vi "Move_Trav_while_Meas_Blocks.vi"() -> (5 "Plug in titles":string[](array[string]), 7 "Plug in values":string[](array[string]))   [LabVIEW 2022 SP3]
uses:
  Controls/Post_Process.ctl
  Controls/Setup.ctl
  Gen Trav/Trav_mode.ctl
  Controls/User_Specific_mode.ctl
  Controls/Tunnel_Coordinates.ctl
  Globals/Trav_pos_global.vi
  Globals/Meas_global.vi
panel:
  in  "2nd delay":u32=6000
  out "Speed Factor":sgl=2.0 min=0.01 max=15 format="%.2f"
  in  "Delay between Rendezvous and Acquisition starting (ms)":u32
  in  "1st delay":u32=2000
  out "Case Currently On":string="Reset Traverse Speed Factor"
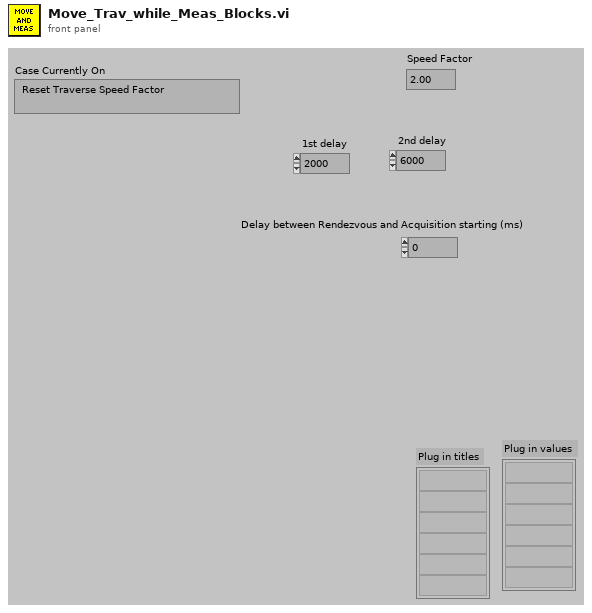
[diagram p1: front panel]
types:
  T1 = typedef "Traverse_cluster.ctl" = cluster{"Start X":sgl, "Start Y":sgl, "Start Z":sgl, "End X":sgl, "End Y":sgl, "End Z":sgl, "nPoints":i32, "Spacing":T2, "Filename":path, "Tunnel Speed":dbl, "Averaging time (mins)":dbl, "Extra Commands":string, "Carrier_1 Q (l/min)":dbl, "Carrier_2 Q (l/min)":dbl, "Trace Gas Concentration (%)":dbl, "Specific Arguments":string, "Comments":string, "Row No":i32, "Row Type Selector":T3, "EstCompl":string, "Row Duration (mins)":dbl, "nValidPoints":i32, "Meas Setup File":string}
  T2 = typedef "Spacing.ctl" = enum16{"Linear", "Log", "Gauss", "Specified", "N/A"}
  T3 = typedef "Multi_run_mode.ctl" = enum16{"Move Traverse Only", "Set Tunnel Speed Only", "Set Source Only", "Set Measurement Conditions", "Single Measurement", "Vertical Profile", "Lateral Profile", "Longitudinal Profile", "Multi-Axis Profile", "Explore Volume", "Auto Calibrate", "Meas Fast FID Bkgnd", "Check Beam Power", "Scanning Valve Measurement", "Run VI Named:", "Set ADAM Ch", "Wait (minutes)", "Send Message", "Synchronize With:", "Fall Back to this Row", "Turn Off Row Repeating", "Traverse 3D Volume", "Blank Row", "Jump to Fall Back Row"}
  T4 = typedef "Setup.ctl" = enum16{"Run Program", "Show Setup", "Save Current Setup", "Setup Front Panel"}
  T5 = typedef "Post_Process.ctl" = enum16{"Take New Data", "Post Process Raw Data File"}
  T6 = typedef "Tunnel_Coordinates.ctl" = enum16{"Work in Tunnel Coordinates", "Work in Model Coordinates"}
  T7 = typedef "User_Specific_mode.ctl" = enum16{"Check VI only", "Run VI"}
  T8 = typedef "Trav_mode.ctl" = enum16{"Move traverse", "Read traverse position", "Teach Position"}
  T9 = typedef "Rendezvous RefNum" = refnum<k1>
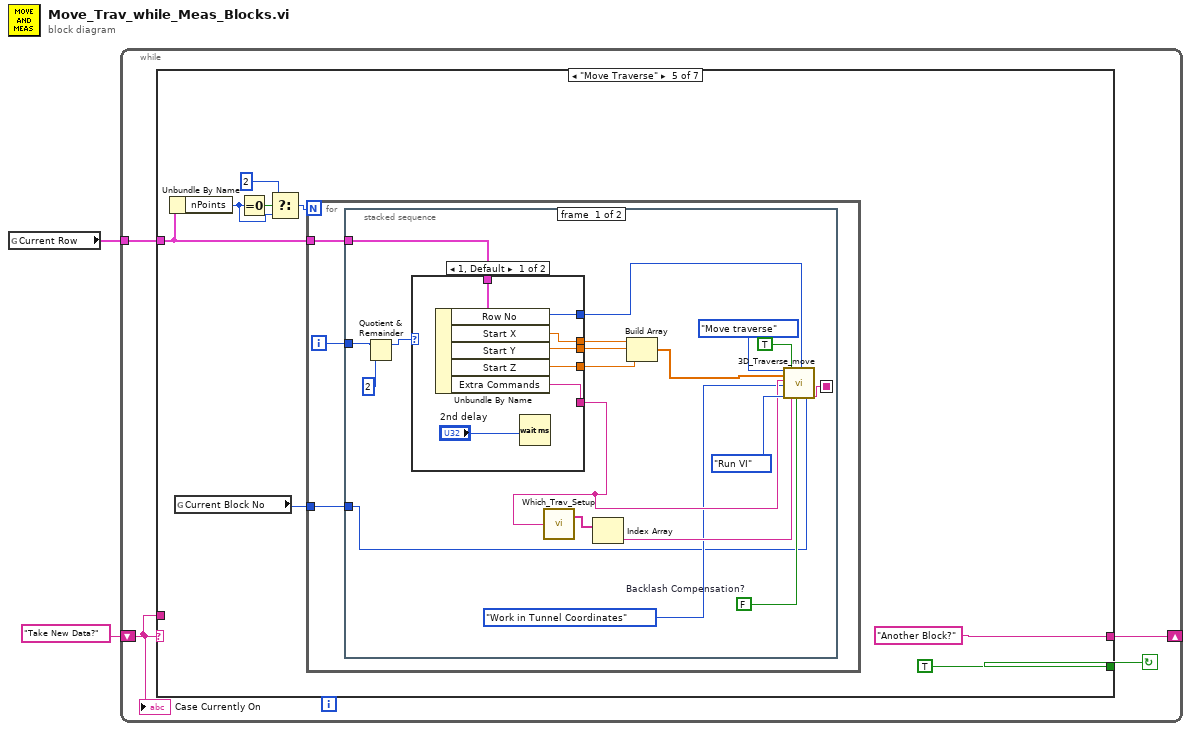
[diagram p0: block diagram]
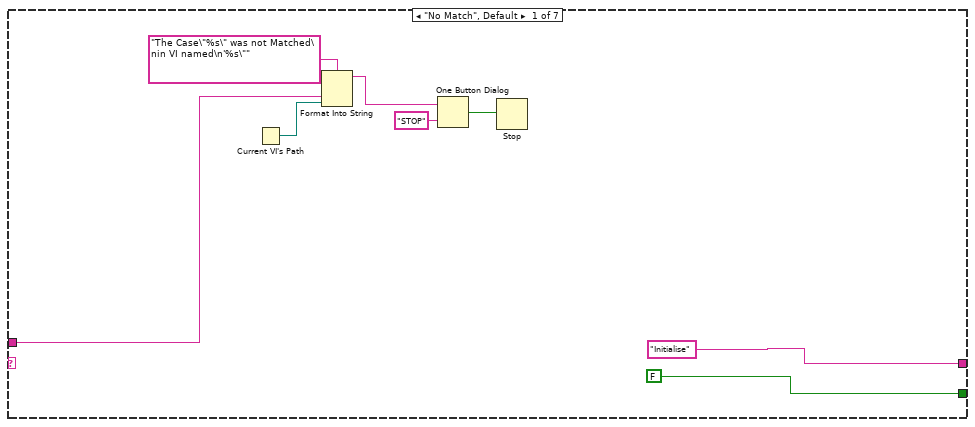
[diagram p2: hidden frame]
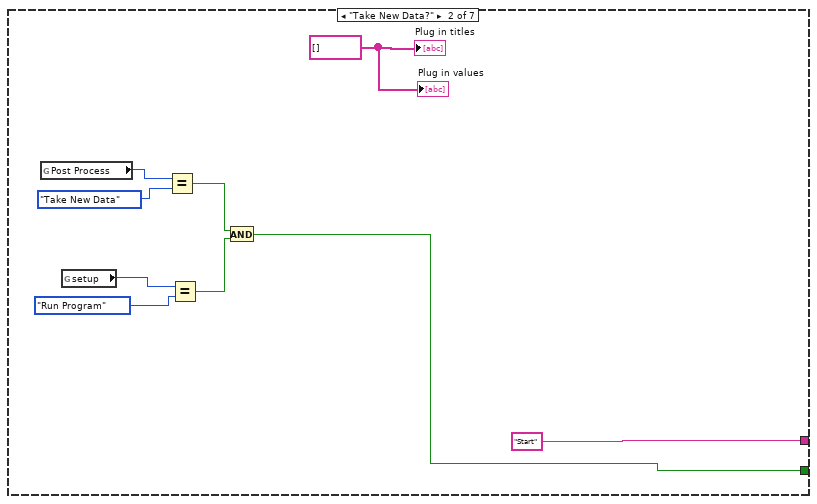
[diagram p3: hidden frame]
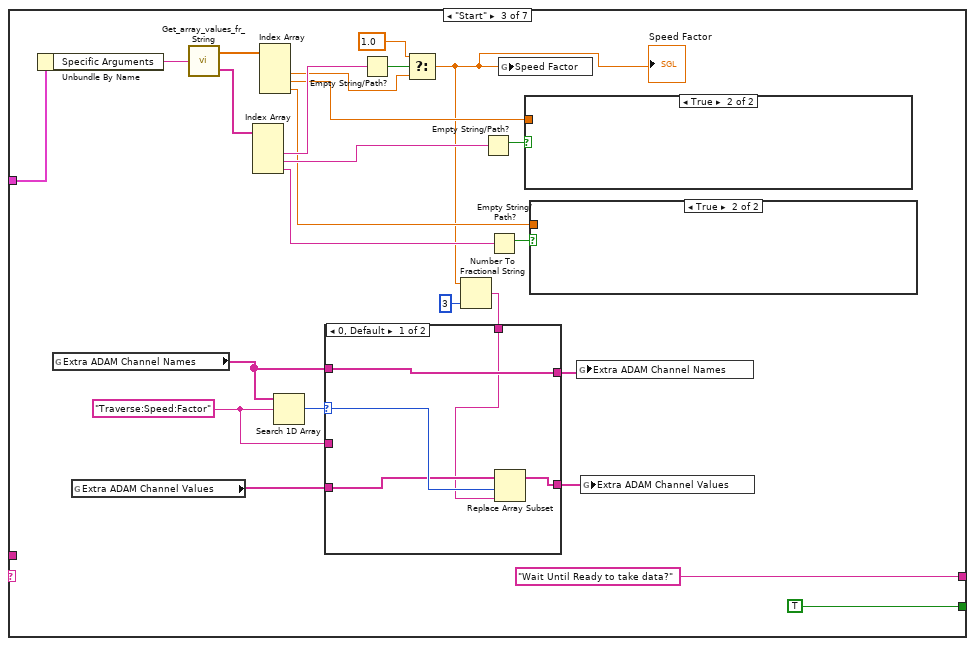
[diagram p4: hidden frame]
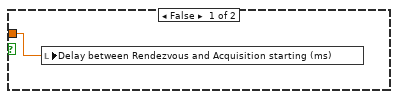
[diagram p5: hidden frame]
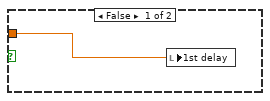
[diagram p6: hidden frame]
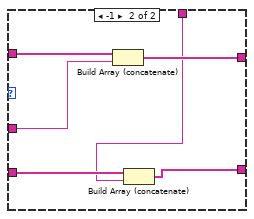
[diagram p7: hidden frame]
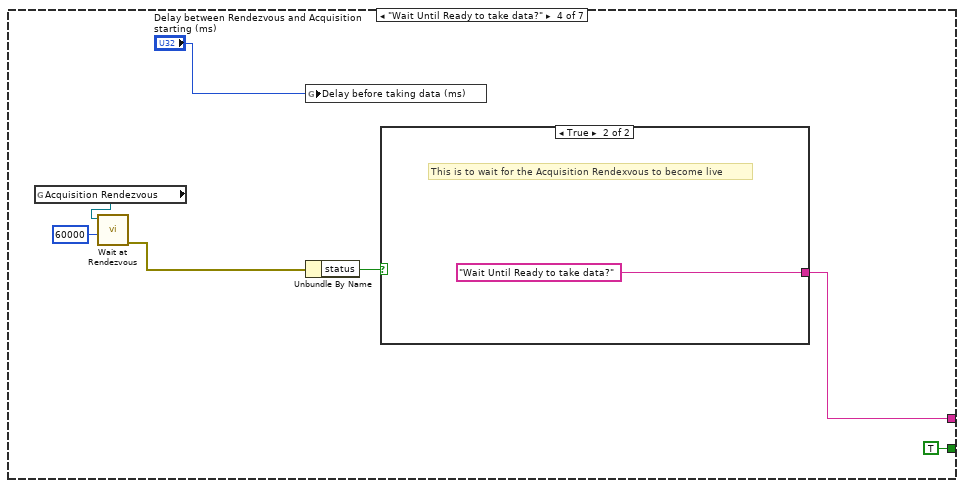
[diagram p8: hidden frame]
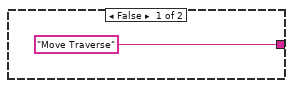
[diagram p9: hidden frame]
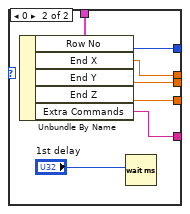
[diagram p10: hidden frame]
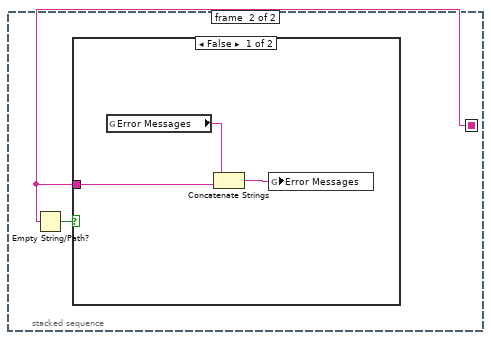
[diagram p11: hidden frame]
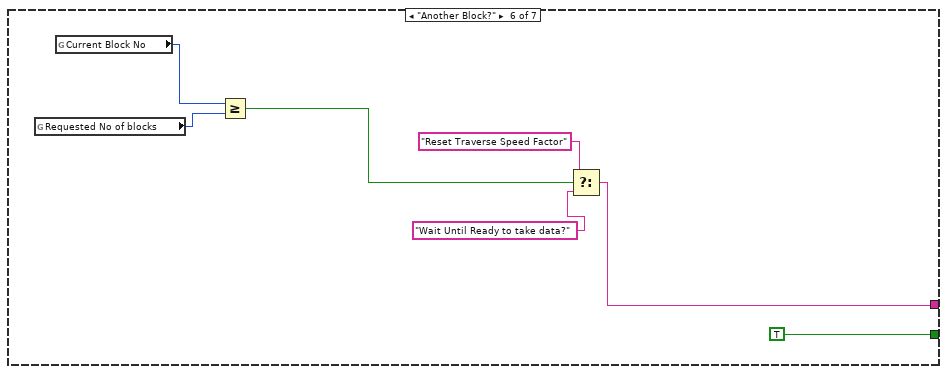
[diagram p13: hidden frame]
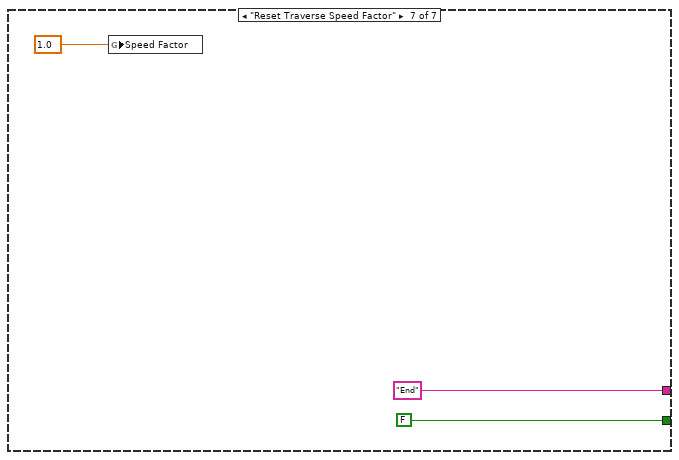
[diagram p14: hidden frame]
diagram:
  n1 = global read "Trav_pos_global.vi" "Current Row"() -> (w1:T1)
  n2 = while {
    shift-left: "Take New Data?" -> [w4]
    shift-right: [w5] -> _
    tunnel: w1 -> [w3]
    stop <- w6 continue-if-true
    n3 = case shown="\"Move Traverse\"" w4 {
      tunnel: [FALSE w15 TRUE ("Command Found") TRUE ("Command Found") TRUE ("Command Found") TRUE ("Command Found") FALSE ("Command Found")] -> w6
      tunnel: ["Initialise" "Start" "Wait Until Ready to take data?" ("f") w64 "Another Block?" w122 "End" ("f")] -> w5
      tunnel: w4 -> [w9 _ _ _ _ _ _]
      tunnel: w3 -> [_ _ w46 _ w75 _ _]
      frame "No Match", Default {
        n4 = Current VI's Path() -> (path=w8:path)
        n5 = Format Into String(format string="The Case\"%s\" was not Matched\nin VI named\n'%s\"" ("Format String"), w9, w8) -> (resulting string=w12:string)  [unwired: 2 in, 1 out]
        n6 = One Button Dialog(message=w12, button name ("OK")="STOP") -> (true=w10:bool)
        n7 = Stop(stop? (T)=w10) -> ()
      }
      frame "Take New Data?" {
        w20 = string[] [] ("Plug in titles")
        n8 = global read "Meas_global.vi" "Post Process"() -> (w22:T5)
        n9 = global read "Meas_global.vi" "setup"() -> (w19:T4)
        n10 = Equal?(x=w22, y=Post_Process."Take New Data" ("Post Process")) -> (x = y?=w16:bool)
        n11 = Equal?(x=w19, y=Setup."Run Program" ("setup")) -> (x = y?=w17:bool)
        n12 = And(x=w16, y=w17) -> (x .and. y?=w15:bool)
        "Plug in titles" <- w20
        "Plug in values" <- w20
      }
      frame "Start" {
        w36 = "Traverse:Speed:Factor"
        n13 = Unbundle By Name(w46) -> ("Specific Arguments"=w48:string)
        n14 = global read "Meas_global.vi" "Extra ADAM Channel Names"() -> (w37:string[])
        n15 = global read "Meas_global.vi" "Extra ADAM Channel Values"() -> (w34:string[])
        n16 = call "Get_array_values_fr_String.vi"("String Value"=w48) -> ("Numeric Array"=w47:dbl[], "String array"=w45:string[])
        n17 = Index Array(array=w45) -> (element #2=w44:string, element #3=w31:string, element #4=w27:string)  [unwired: 4 in, 1 out]
        n18 = Index Array(array=w47) -> (element #2=w42:dbl, element #3=w29:dbl, element #4=w25:dbl)  [unwired: 4 in, 1 out]
        n19 = Search 1D Array(1D array=w37, element=w36) -> (index of element=w38:i32)  [unwired: 1 in]
        n20 = Empty String/Path?(string/path=w44) -> (empty?=w43:bool)
        n21 = Select(t=1.0, s=w43, f=w42) -> (s? t:f=w24:dbl)
        "Speed Factor" <- w24
        n22 = Number To Fractional String(number=w24, precision (6)=i16 3) -> (F-format string=w28:string)  [unwired: 2 in]
        n23 = case shown="0, Default" w38 {
          selector: w38 -> [w54 _]
          tunnel: w37 -> [w55 w61]
          tunnel: w36 -> [_ w60]
          tunnel: [w55 w59] -> w35
          tunnel: w34 -> [w53 w58]
          tunnel: [w52 w57] -> w33
          tunnel: w28 -> [w51 w56]
          frame 0, Default {
            n24 = Replace Array Subset(array=w53, new element=w51, index=w54) -> (w52:string[])
          }
          frame -1 {
            n25 = Build Array (concatenate)(w61, w60) -> (w59:string[])
            n26 = Build Array (concatenate)(w58, w56) -> (w57:string[])
          }
        }
        n27 = Empty String/Path?(string/path=w31) -> (empty?=w30:bool)
        n28 = Empty String/Path?(string/path=w27) -> (empty?=w26:bool)
        n29 = global write "Trav_pos_global.vi" "Speed Factor"(w24) -> ()
        n30 = case shown="True" w30 {
          tunnel: w29 -> [w50 _]
          frame False {
            n31 = local write "1st delay"(w50) -> ()
          }
          frame True {
          }
        }
        n32 = case shown="True" w26 {
          tunnel: w25 -> [w49 _]
          frame False {
            n33 = local write "Delay between Rendezvous and Acquisition starting (ms)"(w49) -> ()
          }
          frame True {
          }
        }
        n34 = global write "Meas_global.vi" "Extra ADAM Channel Names"(w35) -> ()
        n35 = global write "Meas_global.vi" "Extra ADAM Channel Values"(w33) -> ()
      }
      frame "Wait Until Ready to take data?" {
        n36 = global read "Meas_global.vi" "Acquisition Rendezvous"() -> (w67:T9)
        n37 = call <vilib>:"Wait at Rendezvous.vi"("ms timeout (-1)"=60000, "rendezvous"=w67) -> ("error out"=w66:errorcluster)  [unwired: 3 in, 2 out]
        n38 = global write "Meas_global.vi" "Delay before taking data (ms)"("Delay between Rendezvous and Acquisition starting (ms)") -> ()
        n39 = Unbundle By Name(w66) -> ("status"=w63:bool)
        n40 = case shown="True" w63 {
          tunnel: ["Move Traverse" "Wait Until Ready to take data?"] -> w64
          frame False {
          }
          frame True {
            # "This is to wait for the Acquisition Rendexvous to become live"
          }
        }
      }
      frame "Move Traverse" {
        n41 = Unbundle By Name(w75) -> ("nPoints"=w72:i32)
        n42 = global read "Meas_global.vi" "Current Block No"() -> (w76:i32)
        n43 = Equal To 0?(x=w72) -> (x = 0?=w74:bool)
        n44 = Select(t=2, s=w74, f=w72) -> (s? t:f=w73:i32)
        n45 = for {
          N: w73 -> [_]
          tunnel: w75 -> [w81]
          tunnel: w76 -> [w80]
          i -> [w79]
          n46 = stacked-sequence {
            seq-local: [w85 _] -> [_ w115]
            tunnel: w81 -> [w92 _]
            tunnel: w80 -> [w86 _]
            tunnel: w79 -> [w83 _]
            frame #0 {
              w100 = FALSE  # Backlash Compensation?
              n47 = Quotient & Remainder(x=w83, y=2) -> (x-y*floor(x/y)=w82:i32)  [unwired: 1 out]
              n48 = case shown="1, Default" w82 {
                tunnel: [w107 w114] -> w98
                tunnel: [w106 w113] -> w97
                tunnel: [w105 w112] -> w96
                tunnel: [w104 w111] -> w93
                tunnel: w92 -> [w103 w110]
                tunnel: [w102 w109] -> w89
                frame 1, Default {
                  n49 = Unbundle By Name(w103) -> ("Row No"=w104:i32, "Start X"=w107:sgl, "Start Y"=w106:sgl, "Start Z"=w105:sgl, "Extra Commands"=w102:string)
                  n50 = Wait (ms)(milliseconds to wait="2nd delay") -> ()  [unwired: 1 out]
                }
                frame 0 {
                  n51 = Unbundle By Name(w110) -> ("Row No"=w111:i32, "End X"=w114:sgl, "End Y"=w113:sgl, "End Z"=w112:sgl, "Extra Commands"=w109:string)
                  n52 = Wait (ms)(milliseconds to wait="1st delay") -> ()  [unwired: 1 out]
                }
              }
              n53 = call "Which_Trav_Setup.vi"("Extra Command String"=w89) -> ("Traverse Setups"=w91:string[])  [unwired: 2 out]
              n54 = Index Array(array=w91) -> (element=w90:string)  [unwired: 1 in]
              n55 = Build Array(w98, w97, w96) -> (w99:sgl[])
              n56 = call "3D_Traverse_move.vi"("Mode"=Trav_mode."Move traverse", "Position"=w99, "Extra command String"=w89, "Work in Tunnel Coordinates"=Tunnel_Coordinates."Work in Tunnel Coordinates", "Simulate/Run"=User_Specific_mode."Run VI", "Route Checking?"=TRUE, "Traverse name"=w90, "Backlash Compensation?"=w100, "Row Number"=w93, "Currently on Point"=w86) -> ("Error String"=w85:string)  [unwired: 6 in, 3 out]
            }
            frame #1 {
              n57 = Empty String/Path?(string/path=w115) -> (empty?=w116:bool)
              n58 = case shown="False" w116 {
                tunnel: w115 -> [w118 _]
                frame False {
                  n59 = global read "Meas_global.vi" "Error Messages"() -> (w119:string)
                  n60 = Concatenate Strings(w119, w118) -> (w117:string)
                  n61 = global write "Meas_global.vi" "Error Messages"(w117) -> ()
                }
                frame True {
                }
              }
            }
          }
        }
      }
      frame "Another Block?" {
        n62 = global read "Meas_global.vi" "Requested No of blocks"() -> (w126:i32)
        n63 = global read "Meas_global.vi" "Current Block No"() -> (w120:i32)
        n64 = Greater Or Equal?(x=w120, y=w126) -> (x >= y?=w124:bool)
        n65 = Select(t="Reset Traverse Speed Factor", s=w124, f="Wait Until Ready to take data?") -> (s? t:f=w122:string)
      }
      frame "Reset Traverse Speed Factor" {
        n66 = global write "Trav_pos_global.vi" "Speed Factor"(sgl 1.0 ("Speed Factor")) -> ()
      }
    }
    "Case Currently On" <- w4
  }
